vi "Handle Attendance.vi"() -> ()   [LabVIEW 2015, in "Admin_Actor.lvlib"]
uses:
  Admin_Actor.lvlib
  CalAttendance/Type Definitions/NumOfAttendace.ctl
  CalAttendance/Type Definitions/Sign_Attendance.ctl
  CalAttendance/Type Definitions/Main Ctls and VI Refs.ctl
  CalAttendance/CalAttendance.lvclass
  <vilib>/Utility/error.llb/Error Cluster From Error Code.vi
  Setting/g_setting.vi
  <vilib>/ErrorRing/Error Ring.xnode
panel:
  in  "RenewGroup":bool
  out "Sign_Attendance":T1
  out "Num_Attendance":T2
  in  "周次":i32
  in  "组别":string(combo)
  in  "姓名":string(combo)
  in  "Path":path
  in  "Stop":bool
  in  "Save":bool
  in  "Import":bool
  in  "schedule":cluster{"BackGround":u32, "Reason":string}[][](array[cluster])
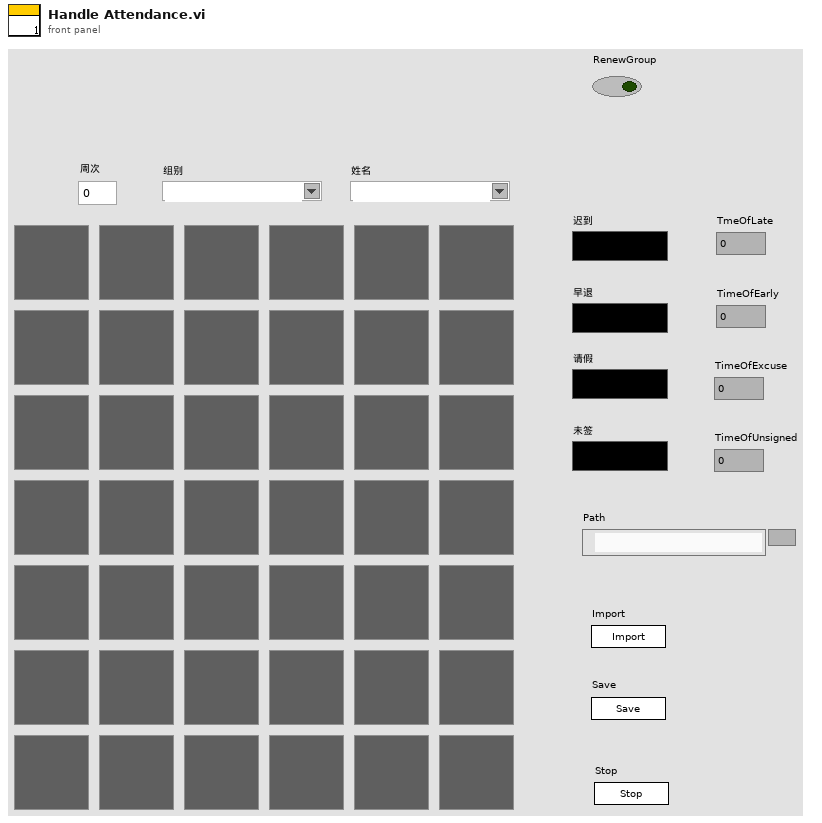
[diagram p1: front panel]
types:
  T1 = typedef "Admin_Actor.lvlib/CalAttendance.lvclass/Sign_Attendance.ctl" = cluster{"早退":u32, "迟到":u32, "请假":u32, "未签":u32}
  T2 = typedef "Admin_Actor.lvlib/CalAttendance.lvclass/NumOfAttendace.ctl" = cluster{"TmeOfLate":i32, "TimeOfEarly":i32, "TimeOfExcuse":i32, "TimeOfUnsigned":i32}
  T3 = typedef "Admin_Actor.lvlib/CalAttendance.lvclass/Main Ctls and VI Refs.ctl" = cluster{"Num_Attendance":refnum<vi>, "Sign_Attendance":refnum<vi>, "Path":refnum<vi>, "周次":refnum<vi>, "姓名":refnum<vi>, "组别":refnum<vi>, "schedule":refnum<vi>, "VI Refnum":refnum<vi>}
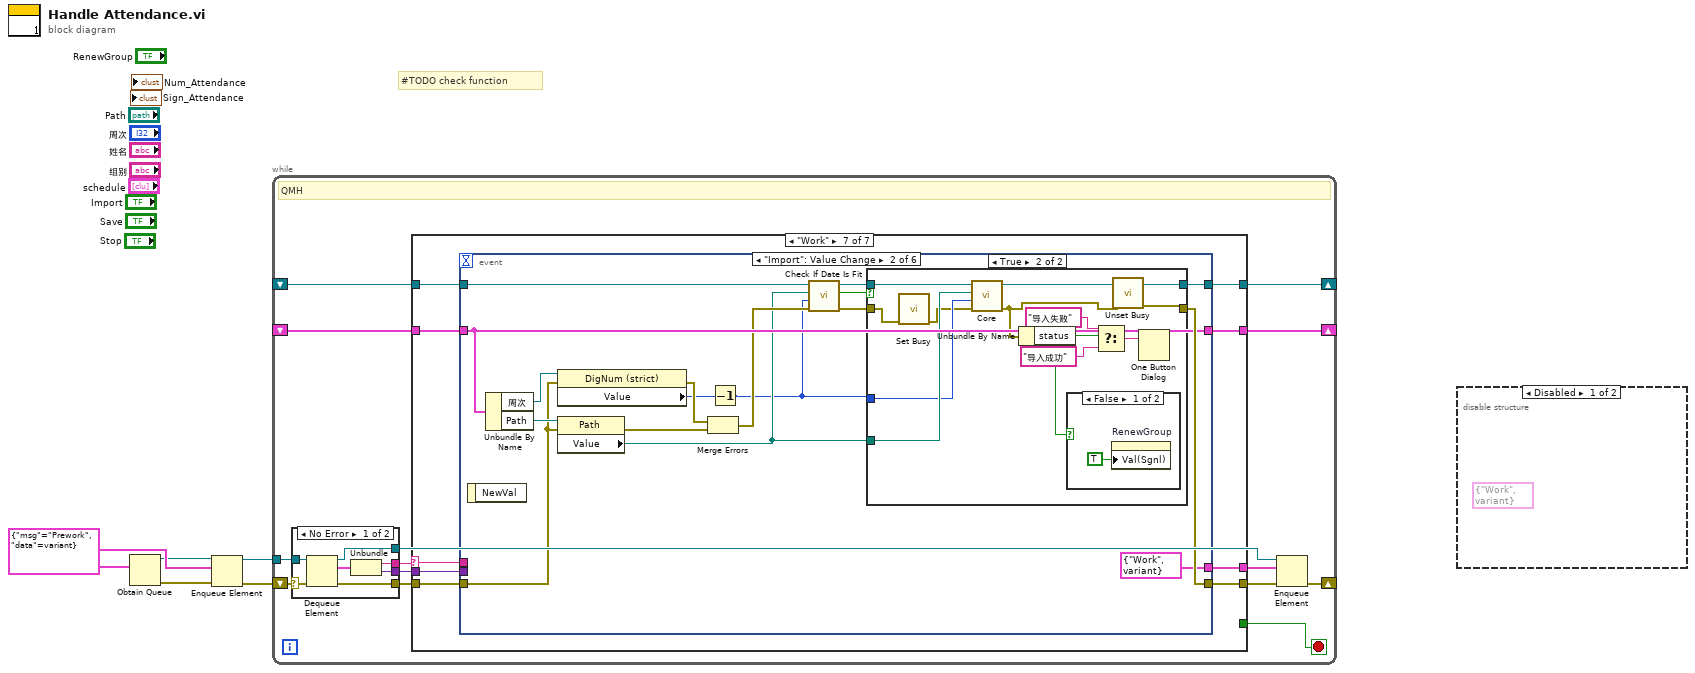
[diagram p0: block diagram]
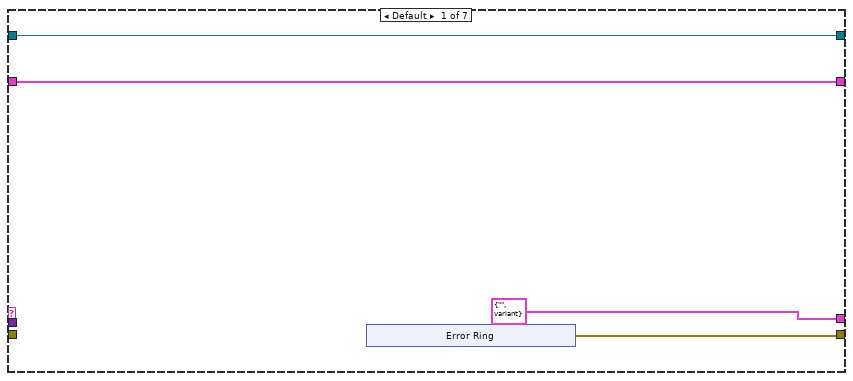
[diagram p3: hidden frame]
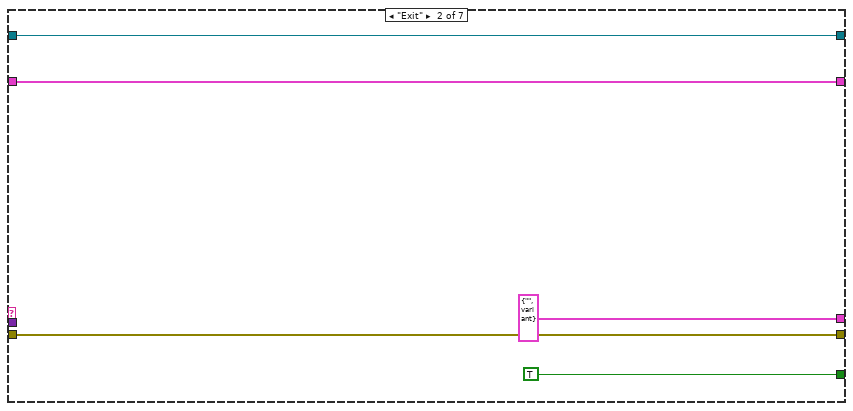
[diagram p4: hidden frame]
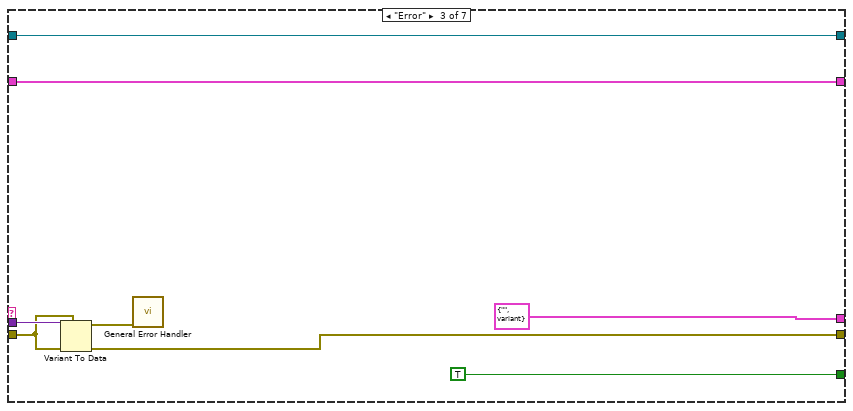
[diagram p5: hidden frame]
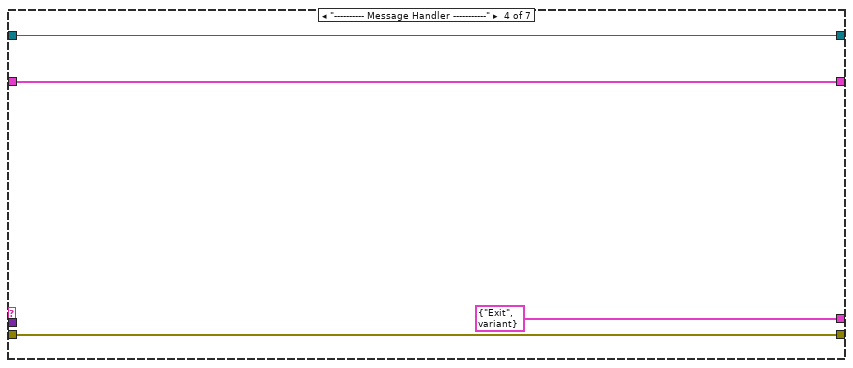
[diagram p6: hidden frame]
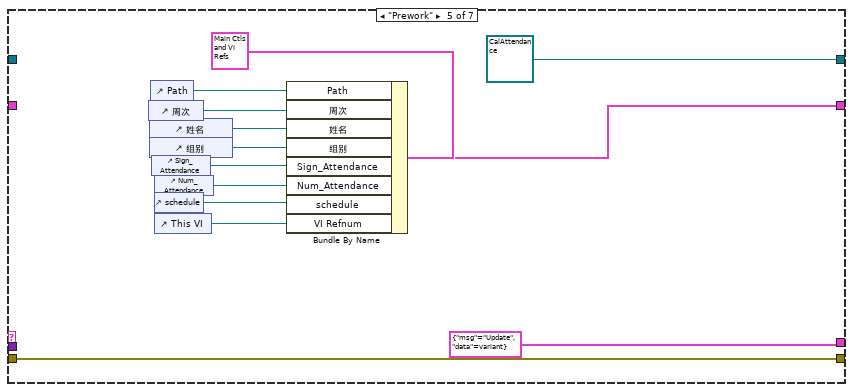
[diagram p7: hidden frame]
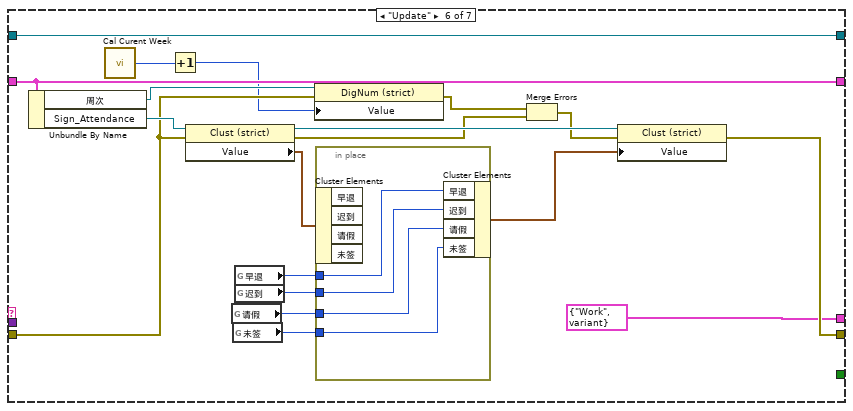
[diagram p8: hidden frame]
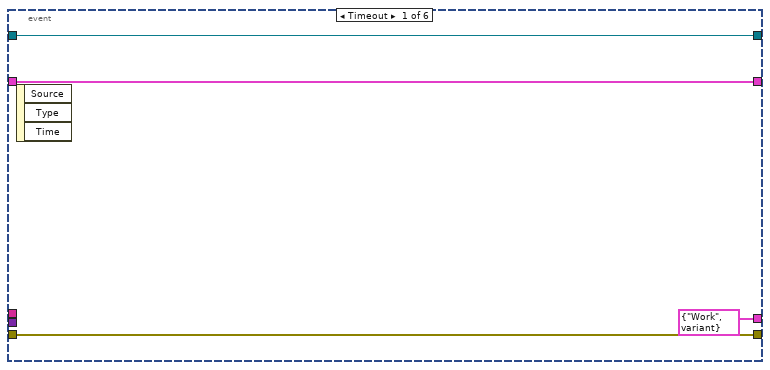
[diagram p9: hidden frame]
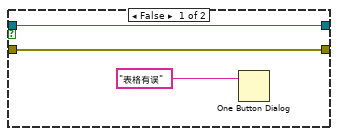
[diagram p10: hidden frame]
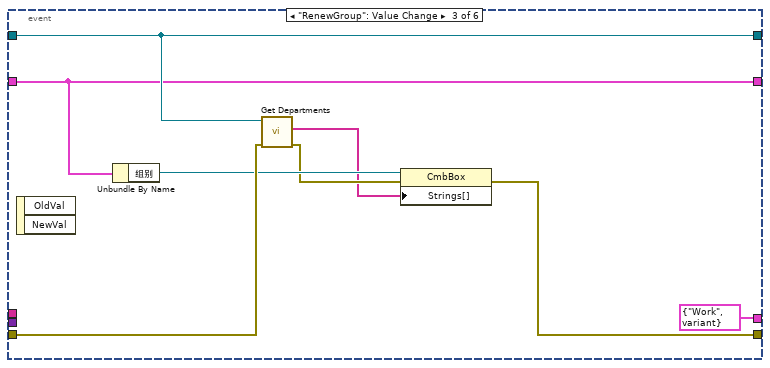
[diagram p12: hidden frame]
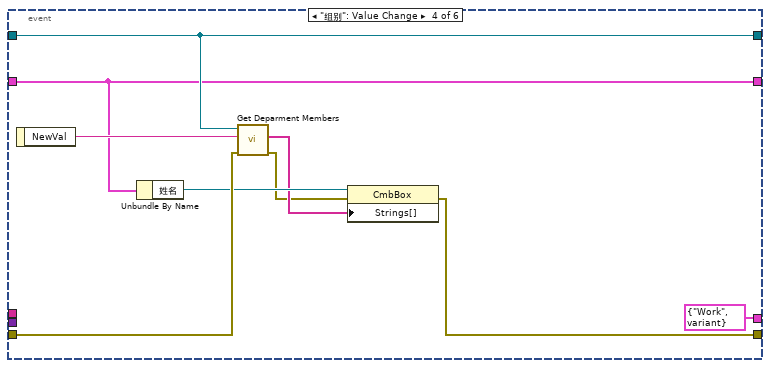
[diagram p13: hidden frame]
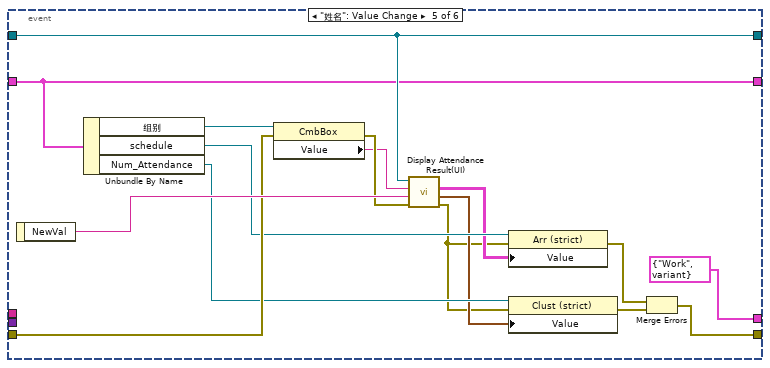
[diagram p14: hidden frame]
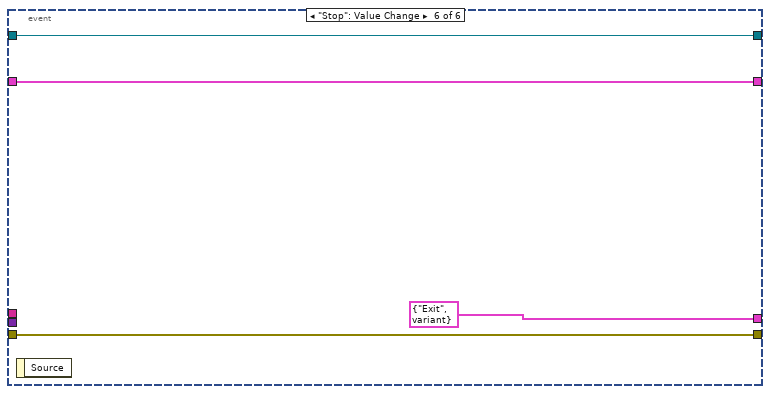
[diagram p15: hidden frame]
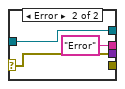
[diagram p16: hidden frame]
diagram:
  w3 = cluster{"msg":string, "data":variant} {"msg"="Prework", "data"=variant}
  # "#TODO check function"
  n1 = Obtain Queue(element data type=w3) -> (queue out=w1:refnum<queue>, error out=w2:errorcluster)  [unwired: 4 in, 1 out]
  n2 = Enqueue Element(queue=w1, element=w3, error in (no error)=w2) -> (queue out=w4:refnum<queue>, error out=w5:errorcluster)  [unwired: 1 in, 1 out]
  n3 = while {
    tunnel: w4 -> [w18]
    shift-right: [w13] -> _
    shift-left: w5 -> [w19]
    shift-right: [w9] -> _
    shift-left: _ -> [w8]
    shift-right: [w7] -> _
    shift-left: _ -> [w6]
    stop <- w10 stop-if-true
    # "QMH"
    n4 = case shown="No Error" w19 {
      selector: w19 -> [w170 w174]
      tunnel: w18 -> [w171 w172]
      tunnel: [w169 _] -> w17
      tunnel: [w167 "Error" ("msg")] -> w16
      tunnel: [w166 w174] -> w15
      tunnel: [w165 w172] -> w12
      frame No Error {
        n5 = Dequeue Element(queue=w171, error in (no error)=w170) -> (queue out=w165:refnum<queue>, element=w168:cluster{"msg":string, "data":variant}, error out=w169:errorcluster)  [unwired: 1 in, 1 out]
        n6 = Unbundle(w168) -> ("msg"=w167:string, "data"=w166:variant)
      }
      frame Error {
      }
    }
    n7 = case shown="\"Work\"" w16 {
      selector: w16 -> [_ _ _ _ _ _ w88]
      tunnel: w17 -> [_ w33 w40 w45 w57 w64 w90]
      tunnel: w15 -> [_ _ w41 _ _ _ w89]
      tunnel: [w23 w33 w38 w45 w57 w71 w87] -> w14
      tunnel: [cluster{"msg":string, "data":variant} {"msg"="", "data"=variant} cluster{"msg":string, "data":variant} {"msg"="", "data"=variant} cluster{"msg":string, "data":variant} {"msg"="", "data"=variant} cluster{"msg":string, "data":variant} {"msg"="Exit", "data"=variant} cluster{"msg":string, "data":variant} {"msg"="Update", "data"=variant} cluster{"msg":string, "data":variant} {"msg"="Work", "data"=variant} w86] -> w11
      tunnel: [_ TRUE TRUE _ _ _ _] -> w10
      tunnel: [w20 w29 w34 w42 w55 w76 w82] -> w9
      tunnel: w8 -> [w20 w29 w34 w42 _ w76 w84]
      tunnel: [w21 w30 w35 w43 refnum<class "CalAttendance.lvclass"> refnum ("Admin_Actor.lvlib:CalAttendance.lvclass") w77 w83] -> w7
      tunnel: w6 -> [w21 w30 w35 w43 _ w77 w85]
      frame Default {
        n8 = xnode ("Error Ring")() -> ("error out"=w23:errorcluster)
      }
      frame "Exit" {
      }
      frame "Error" {
        n9 = Variant To Data(error in=w40, type=w40, Variant=w41) -> (data=w39:errorcluster, error out=w38:errorcluster)
        n10 = call <vilib>:"General Error Handler.vi"("error in (no error)"=w39) -> ()  [unwired: 10 in, 5 out]
      }
      frame "---------- Message Handler -----------" {
      }
      frame "Prework" {
        n11 = control-ref of="周次"() -> (w54:refnum<vi>)
        n12 = control-ref of="姓名"() -> (w53:refnum<vi>)
        n13 = control-ref of="组别"() -> (w52:refnum<vi>)
        n14 = control-ref of="Path"() -> (w50:refnum<vi>)
        n15 = control-ref of="Sign_Attendance"() -> (w49:refnum<vi>)
        n16 = control-ref of="Num_Attendance"() -> (w48:refnum<vi>)
        n17 = control-ref of="schedule"() -> (w47:refnum<vi>)
        n18 = control-ref of="This VI"() -> (w46:refnum<vi>)
        n19 = Bundle By Name(cluster=T3 {"Num_Attendance"=refnum, "Sign_Attendance"=refnum, "Path"=refnum, "周次"=refnum, "姓名"=refnum, "组别"=refnum, "schedule"=refnum, "VI Refnum"=refnum} ("Refs"), "Path"=w50, "周次"=w54, "姓名"=w53, "组别"=w52, "Sign_Attendance"=w49, "Num_Attendance"=w48, "schedule"=w47, "VI Refnum"=w46) -> (w55:T3)
      }
      frame "Update" {
        n20 = Unbundle By Name(w76) -> ("周次"=w65:refnum<vi>, "Sign_Attendance"=w75:refnum<vi>)
        n21 = call "Cal Curent Week.vi"() -> ("CurWeek(0)"=w60:i32)
        n22 = Increment(x=w60) -> (x+1=w59:i32)
        n23 = property class="Clust (strict)"(reference=w75, error in=w64) -> (reference out=w73:refnum<vi>, error out=w62:errorcluster, "Value"=w74:cluster{"早退":u32, "迟到":u32, "请假":u32, "未签":u32})
        n24 = global read "g_setting.vi" "请假"() -> (w67:u32)
        n25 = global read "g_setting.vi" "未签"() -> (w66:u32)
        n26 = global read "g_setting.vi" "早退"() -> (w69:u32)
        n27 = global read "g_setting.vi" "迟到"() -> (w68:u32)
        n28 = property class="DigNum (strict)"(reference=w65, error in=w64, "Value"=w59) -> (error out=w63:errorcluster)  [unwired: 1 out]
        n29 = in-place {
          in-place-border: w69 -> [w81]
          in-place-border: w68 -> [w80]
          in-place-border: w67 -> [w79]
          in-place-border: w66 -> [w78]
          n30 = in-place-cluster #1(w74) -> ()  [unwired: 4 out]
          n31 = in-place-cluster #1("早退"=w81, "迟到"=w80, "请假"=w79, "未签"=w78) -> (w72:cluster{"早退":u32, "迟到":u32, "请假":u32, "未签":u32})
        }
        n32 = Merge Errors(w63, w62) -> (w61:errorcluster)
        n33 = property class="Clust (strict)"(reference=w73, error in=w61, "Value"=w72) -> (error out=w71:errorcluster)  [unwired: 1 out]
      }
      frame "Work" {
        n34 = event shown="[1] \"Import\": Value Change" {
          selector: _ -> [_ _ _ _ _ _]
          dyn-events: _ -> [_ _ _ _ _ _]
          timeout: _ -> [_ _ _ _ _ _]
          tunnel: w90 -> [w94 w109 w133 w142 w156 w164]
          tunnel: w89 -> [_ _ _ _ _ _]
          tunnel: w88 -> [_ _ _ _ _ _]
          tunnel: [w94 w106 w129 w137 w146 w164] -> w87
          tunnel: [cluster{"msg":string, "data":variant} {"msg"="Work", "data"=variant} cluster{"msg":string, "data":variant} {"msg"="Work", "data"=variant} cluster{"msg":string, "data":variant} {"msg"="Work", "data"=variant} cluster{"msg":string, "data":variant} {"msg"="Work", "data"=variant} cluster{"msg":string, "data":variant} {"msg"="Work", "data"=variant} cluster{"msg":string, "data":variant} {"msg"="Exit", "data"=variant}] -> w86
          tunnel: w85 -> [w92 w103 w135 w144 w160 w162]
          tunnel: w84 -> [w91 w104 w134 w141 w158 w161]
          tunnel: [w92 w105 w135 w144 w160 w162] -> w83
          tunnel: [w91 w104 w134 w141 w158 w161] -> w82
          event Timeout {
            n35 = event-data() -> ()  [unwired: 1 in, 3 out]
          }
          event "Import": Value Change {
            n36 = event-data() -> ()  [unwired: 1 in, 1 out]
            n37 = Unbundle By Name(w104) -> ("周次"=w110:refnum<vi>, "Path"=w111:refnum<vi>)
            n38 = property class="DigNum (strict)"(reference=w110, error in=w109) -> (error out=w108:errorcluster, "Value"=w96:i32)  [unwired: 1 out]
            n39 = property class="Path"(reference=w111, error in=w109) -> (error out=w107:errorcluster, "Value"=w101:path)  [unwired: 1 out]
            n40 = Merge Errors(w108, w107) -> (w102:errorcluster)
            n41 = Decrement(x=w96) -> (x-1=w95:i32)
            n42 = call "Check If Date Is Fit.vi"("error in (no error)"=w102, "CurWeek(0)"=w95, "Path"=w101, "CalAttendance in"=w103) -> ("error out"=w100:errorcluster, "Fit(False)"=w98:bool, "CalAttendance out"=w99:refnum<class "CalAttendance.lvclass">)  [unwired: 5 in]
            n43 = case shown="True" w98 {
              tunnel: [w113 w117] -> w106
              tunnel: [w114 w126] -> w105
              tunnel: w101 -> [_ w125]
              tunnel: w95 -> [_ w124]
              tunnel: w100 -> [w113 w119]
              tunnel: w99 -> [w114 w123]
              frame False {
                n44 = One Button Dialog(message="表格有误") -> ()  [unwired: 1 in, 1 out]
              }
              frame True {
                n45 = call <vilib>:"Set Busy.vi"("error in (no error)"=w119) -> ("error out"=w118:errorcluster)  [unwired: 9 in, 1 out]
                n46 = call "Core.vi"("error in (no error)"=w118, "CurWeek(0)"=w124, "ExcusePath"=w125, "CalAttendance in"=w123) -> ("error out"=w116:errorcluster, "CalAttendance out"=w126:refnum<class "CalAttendance.lvclass">)  [unwired: 6 in]
                n47 = Unbundle By Name(w116) -> ("status"=w115:bool)
                n48 = case shown="False" w115 {
                  frame False {
                    n49 = property on="RenewGroup" class="Bool (strict)"("Val(Sgnl)"=TRUE ("Value (Signaling)")) -> ()  [unwired: 2 in, 2 out]
                  }
                  frame True {
                  }
                }
                n50 = Select(t="导入失败", s=w115, f="导入成功") -> (s? t:f=w120:string)
                n51 = call <vilib>:"Unset Busy.vi"("error in (no error)"=w116) -> ("error out"=w117:errorcluster)  [unwired: 10 in]
                n52 = One Button Dialog(message=w120) -> ()  [unwired: 1 in, 1 out]
              }
            }
          }
          event "RenewGroup": Value Change {
            n53 = event-data() -> ()  [unwired: 1 in, 2 out]
            n54 = Unbundle By Name(w134) -> ("组别"=w132:refnum<vi>)
            n55 = call "Get Departments.vi"("error in (no error)"=w133, "CalAttendance in"=w135) -> ("error out"=w131:errorcluster, "Departments(\"\")"=w130:string[])  [unwired: 7 in, 1 out]
            n56 = property class="CmbBox"(reference=w132, error in=w131, "Strings[]"=w130) -> (error out=w129:errorcluster)  [unwired: 1 out]
          }
          event "组别": Value Change {
            n57 = event-data() -> ("NewVal"=w143:string)  [unwired: 1 in]
            n58 = Unbundle By Name(w141) -> ("姓名"=w140:refnum<vi>)
            n59 = call "Get Deparment Members.vi"("error in (no error)"=w142, "Department(\"\")"=w143, "CalAttendance in"=w144) -> ("error out"=w138:errorcluster, "Names(\"\")"=w139:string[])  [unwired: 6 in, 1 out]
            n60 = property class="CmbBox"(reference=w140, error in=w138, "Strings[]"=w139) -> (error out=w137:errorcluster)  [unwired: 1 out]
          }
          event "姓名": Value Change {
            n61 = event-data() -> ("NewVal"=w159:string)  [unwired: 1 in]
            n62 = Unbundle By Name(w158) -> ("组别"=w157:refnum<vi>, "schedule"=w153:refnum<vi>, "Num_Attendance"=w151:refnum<vi>)
            n63 = property class="CmbBox"(reference=w157, error in=w156) -> (error out=w155:errorcluster, "Value"=w154:string)  [unwired: 1 out]
            n64 = call "Display Attendance Result(UI).vi"("error in (no error)"=w155, "Name(\"\")"=w159, "Department(\"\")"=w154, "CalAttendance in"=w160) -> ("error out"=w149:errorcluster, "NumOfAttendance"=w150:T2, "Res_Attendance"=w152:cluster{"BackGround":u32, "Reason":string}[][])  [unwired: 4 in, 1 out]
            n65 = property class="Arr (strict)"(reference=w153, error in=w149, "Value"=w152) -> (error out=w148:errorcluster)  [unwired: 1 out]
            n66 = property class="Clust (strict)"(reference=w151, error in=w149, "Value"=w150) -> (error out=w147:errorcluster)  [unwired: 1 out]
            n67 = Merge Errors(w148, w147) -> (w146:errorcluster)
          }
          event "Stop": Value Change {
            n68 = event-data() -> ()  [unwired: 1 in, 1 out]
          }
        }
      }
    }
    n69 = Enqueue Element(queue=w12, element=w11, error in (no error)=w14) -> (error out=w13:errorcluster)  [unwired: 1 in, 2 out]
  }
  n70 = disable-structure shown="Disabled" {
    frame Disabled {
      (unwired) cluster{"msg":string, "data":variant} {"msg"="Work", "data"=variant}
    }
    frame Enabled {
    }
  }
